vi "Teleop.vi"(10 "Match Info":T1={"Autonomous Elapsed Seconds"=0.0, "TeleOp Elapsed Seconds"=0.0, "Disabled Elapsed Seconds"=0.0, "Visited Autonomous"=FALSE, "Visited TeleOp"=FALSE, "Visited Disabled"=FALSE, "Autonomous Settings"={"Autonomous Style"=enum."Independent", "VI Refnum"=refnum}}, 11 "Call Context":T2) -> ()   [LabVIEW 2016]
doc: "This VI is called for each TeleOp packet received from the DS where the robot is not disabled. It is often used to read from the joysticks and update I/O or to update setpoints for timed control loops. It should complete and return within 20 milliseconds or it may miss DS packets."
uses:
  <vilib>/Rock Robotics/WPI/DriverStation/WPI_DriverStationDerivedRobotMode.ctl
  <vilib>/Rock Robotics/WPI/DriverStation/WPI_DriverStationMatch Info.ctl
  <vilib>/Rock Robotics/WPI/Solenoid/WPI_SolenoidValue.ctl
  <vilib>/Rock Robotics/WPI/Utilities/WPI_GetSetVariantRefNum.vi
  <vilib>/Rock Robotics/WPI/Solenoid/WPI_SolenoidSetEnum.vi
panel:
  out "Gyro Angle":dbl format="%#_13g"
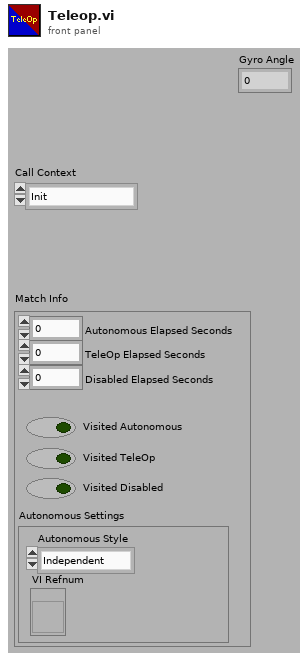
[diagram p1: front panel]
types:
  T1 = typedef "WPI_DriverStationMatch Info.ctl" = cluster{"Autonomous Elapsed Seconds":dbl, "TeleOp Elapsed Seconds":dbl, "Disabled Elapsed Seconds":dbl, "Visited Autonomous":bool, "Visited TeleOp":bool, "Visited Disabled":bool, "Autonomous Settings":cluster{"Autonomous Style":enum16{"Iterative", "Independent"}, "VI Refnum":refnum<vi>}}
  T2 = typedef "WPI_DriverStationDerivedRobotMode.ctl" = enum16{"Init", "Execute", "Stop"}
  T3 = typedef "WPI_SolenoidValue.ctl" = enum16{"Off", "On", "Forward", "Reverse"}
  T4 = typedef "WPI_AccelerometerDevRef.ctl" = cluster{"DevStatus":errorcluster, "Scaling":T5, "Analog Channels":T6, "I2C Bus":T8, "SPI Bus":T9, "Accel Range":T10, "ADXL Axes":T11, "Handle":i32, "Device Address":u8, "Accel Type":enum16{"Analog", "ADXL345 I2C", "ADXL345 SPI", "Internal", "ADXL362 SPI"}}
  T5 = typedef "WPI_AccelerometerScaling.ctl" = cluster{"Gain (VoltsPerG)":dbl, "Center Voltage":dbl}
  T6 = typedef "WPI_AccelerometerAnalogChannels.ctl" = cluster{"X-Axis":T7, "Y-Axis":T7, "Z-Axis":T7}
  T7 = typedef "FPGA_AIChannel.ctl" = enum8{"AI 0", "AI 1", "AI 2", "AI 3", "AI MXP 0", "AI MXP 1", "AI MXP 2", "AI MXP 3", "Invalid"}
  T8 = typedef "i2c_bus.ctl" = enum16{"I2C On-Board", "I2C MXP", "Invalid"}
  T9 = typedef "spi_bus.ctl" = enum16{"SPI On-Board, CS0", "SPI On-Board, CS1", "SPI On-Board, CS2", "SPI On-Board, CS3", "SPI MXP", "Invalid"}
  T10 = typedef "ADXL345 Range.ctl" = u8
  T11 = typedef "WPI_AccelerometerADXL345 Axes.ctl" = cluster{"X-Axis":bool, "Y-Axis":bool, "Z-Axis":bool}
  T12 = cluster{"X-Axis":dbl, "Y-Axis":dbl, "Z-Axis":dbl}
  T13 = typedef "WPI_GyroDevRef.ctl" = cluster{"DevStatus":errorcluster, "Analog Channel":T7, "Offset":dbl, "Gain (VoltsPerDegree/Second)":dbl, "Gyro Type":enum16{"Analog", "XRS450"}, "Handle":i32, "SPI Bus":T9, "Device Found":bool, "Sample Rate":dbl, "Calibrate On Open":bool}
  T14 = typedef "WPI_JoystickDevRef.ctl" = cluster{"Device":T15}
  T15 = typedef "WPI_JoystickDeviceEnum.ctl" = enum16{"USB 0", "USB 1", "USB 2", "USB 3", "USB 4", "USB 5"}
  T16 = typedef "WPI_MotorControlDeviceRef.ctl" = cluster{"DeviceStatus":errorcluster, "Type":T17, "PWM":cluster{"PWM Channel":T18, "DeadBand":T19}, "CAN":cluster{"Device Number":u8, "SetOutput VI Ref":variant, "GetOutput VI Ref":variant, "Enable VI Ref":variant, "Disable VI Ref":variant, "Data":variant}, "Invert":bool}
  T17 = typedef "WPI_MotorControlType.ctl" = enum16{"PWM", "CAN"}
  T18 = typedef "FPGA_DIOPWMChannel.ctl" = enum8{"PWM 0", "PWM 1", "PWM 2", "PWM 3", "PWM 4", "PWM 5", "PWM 6", "PWM 7", "PWM 8", "PWM 9", "PWM MXP 0", "PWM MXP 1", "PWM MXP 2", "PWM MXP 3", "PWM MXP 4", "PWM MXP 5", "PWM MXP 6", "PWM MXP 7", "PWM MXP 8", "PWM MXP 9", "Invalid"}
  T19 = typedef "WPI_PWMDeadband.ctl" = cluster{"Name":string, "maxPositivePwm":i32, "minPositivePwm":i32, "centerPwm":i32, "maxNegativePwm":i32, "minNegativePwm":i32, "angularRange":u16}
  T20 = typedef "WPI_SolenoidDevRef.ctl" = cluster{"DevStatus":errorcluster, "Pneumatics Control Module":u8, "Forward Solenoid Channel":T21, "Reverse Solenoid Channel":T21}
  T21 = typedef "WPI_SolenoidChannel.ctl" = enum8{"Solenoid 0", "Solenoid 1", "Solenoid 2", "Solenoid 3", "Solenoid 4", "Solenoid 5", "Solenoid 6", "Solenoid 7", "Invalid"}
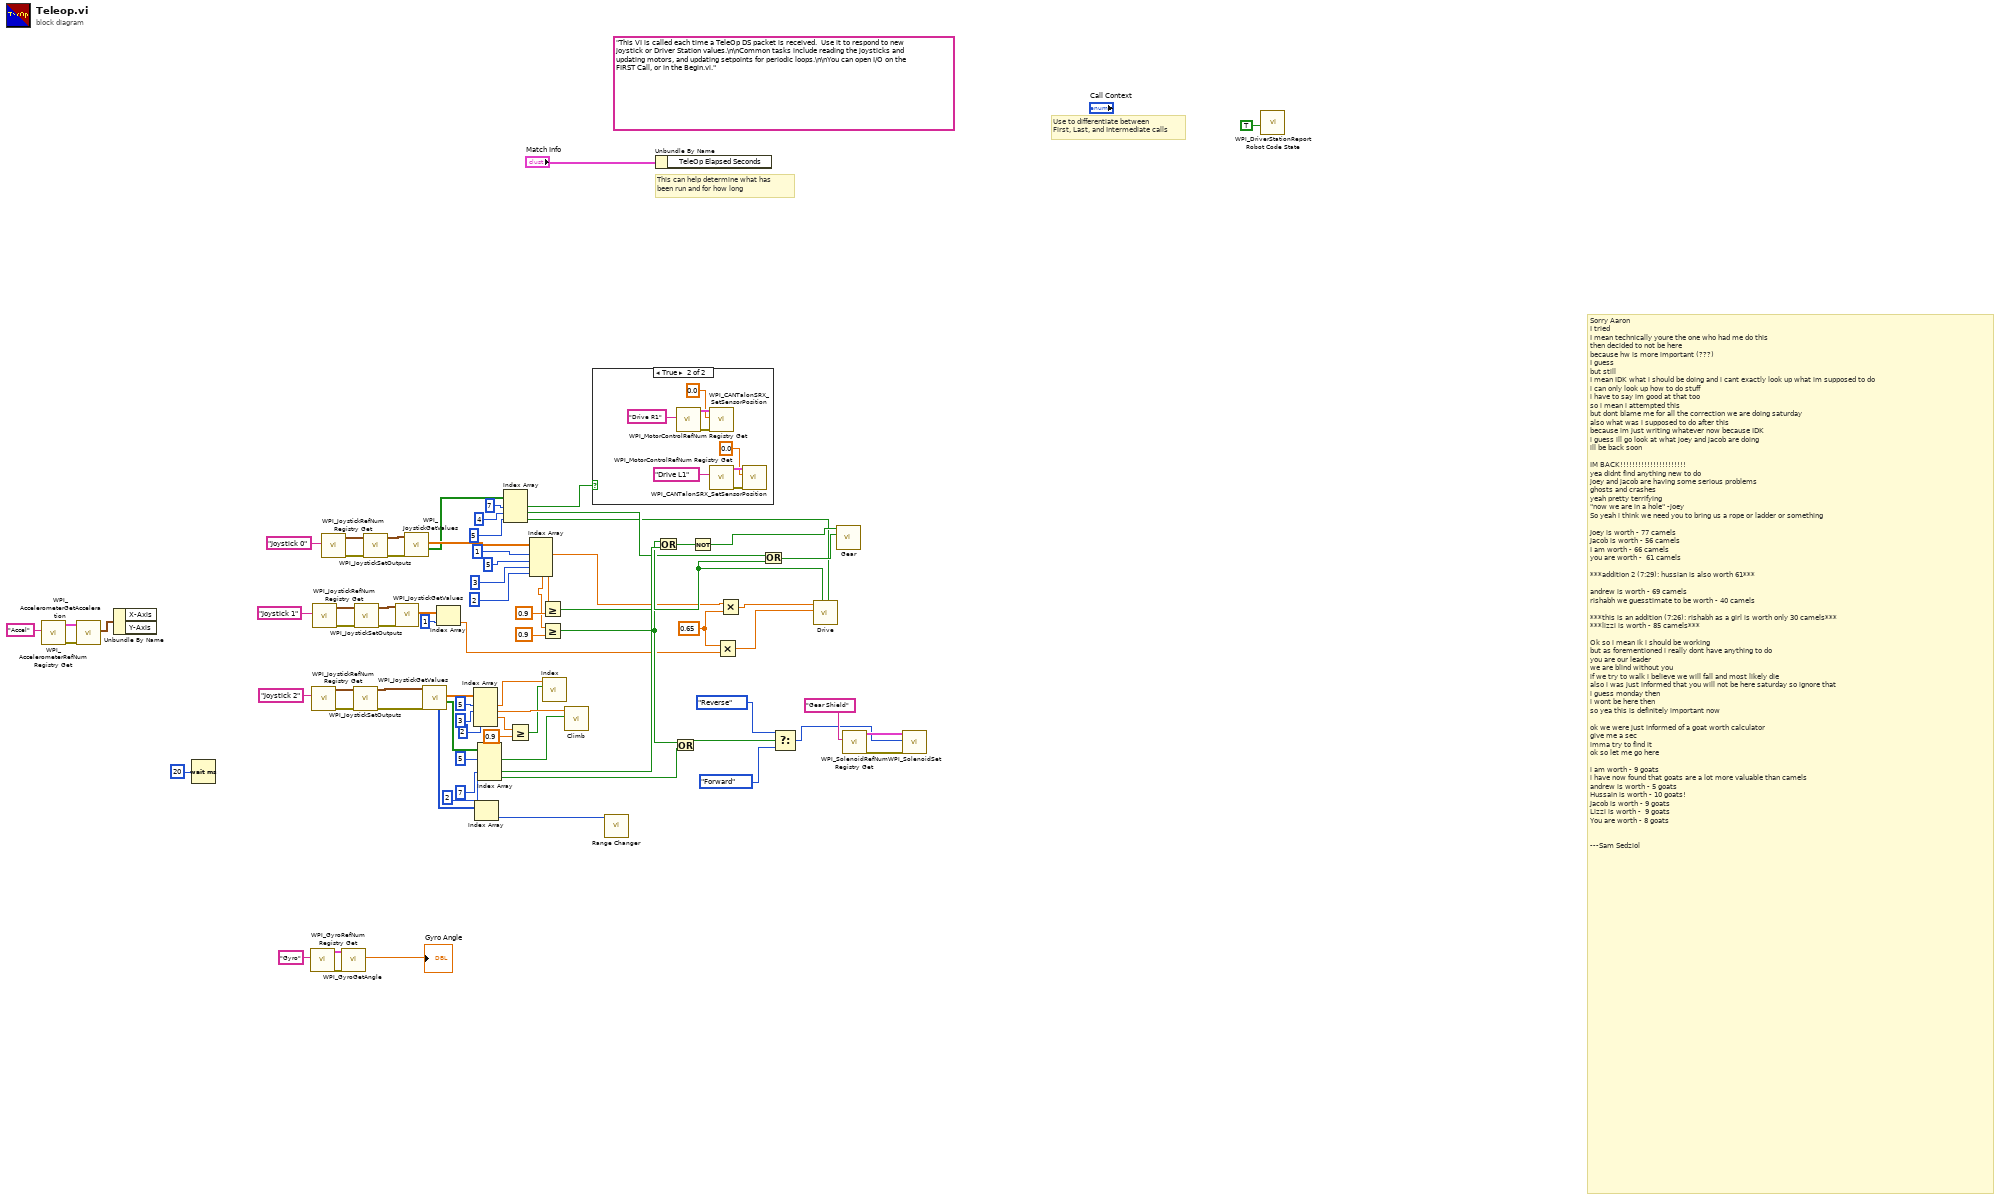
[diagram p0: block diagram]
diagram:
  w1 = 0.65
  (unwired) "This VI is called each time a TeleOp DS packet is received.  Use it to respond to new joystick or Driver Station values.\n\nCommon tasks include reading the joysticks and updating motors, and updating setpoints for periodic loops.\n\nYou can open I/O on the FIRST Call, or in the Begin.vi."
  # "Sorry Aaron\nI tried\nI mean technically youre the one who had me do this\nthen decided to not be here\nbecause hw is more important (???)\nI guess\nbut still\nI mean IDK what i should be doing and i cant exactly look up what im supposed to do\ni can only look up how to do stuff\ni have to say im good at that too\nso i mean i attempted this\nbut dont blame me for all the correction we are doing saturday\nalso what was i supposed to do after this\nbecause im just writing whatever now because IDK\ni guess ill go look at what joey and jacob are doing\nill be back soon\n\nIM BACK!!!!!!!!!!!!!!!!!!!!!!\nyea didnt find anything new to do\njoey and jacob are having some serious problems\nghosts and crashes\nyeah pretty terrifying\n\"now we are in a hole\" -joey\nSo yeah i think we need you to bring us a rope or ladder or something\n\nJoey is worth - 77 camels\nJacob is worth - 56 camels\nI am worth - 66 camels\nyou are worth -  61 camels \n\n***addition 2 (7:29): hussian is also worth 61***\n\nandrew is worth - 69 camels\nrishabh we guesstimate to be worth - 40 camels\n\n***this is an addition (7:26): rishabh as a girl is worth only 30 camels***\n***lizzi is worth - 85 camels***\n\nOk so i mean ik i should be working\nbut as forementioned i really dont have anything to do\nyou are our leader\nwe are blind without you\nif we try to walk i believe we will fall and most likely die\nalso i was just informed that you will not be here saturday so ignore that\ni guess monday then\ni wont be here then\nso yea this is definitely important now\n\nok we were just informed of a goat worth calculator\ngive me a sec \nimma try to find it\nok so let me go here\n\ni am worth - 9 goats\ni have now found that goats are a lot more valuable than camels\nandrew is worth - 5 goats\nHussain is worth - 10 goats! \nJacob is worth - 9 goats\nLizzi is worth -  9 goats\nYou are worth - 8 goats\n\n\n---Sam Sedziol"
  # "Use to differentiate between\nFirst, Last, and Intermediate calls"
  # "This can help determine what has\nbeen run and for how long"
  n1 = call <vilib>:"WPI_AccelerometerRefNum Registry Get.vi"("refnum name"="Accel") -> ("error out"=w23:errorcluster, "AccelerometerDevRef"=w22:T4)  [unwired: 9 in]
  n2 = call <vilib>:"WPI_AccelerometerGetAcceleration.vi"("error in"=w23, "AccelerometerDevRef"=w22) -> ("Accelerations"=w24:T12)  [unwired: 7 in, 2 out]
  n3 = Unbundle By Name(w24) -> ()  [unwired: 2 out]
  n4 = Wait (ms)(milliseconds to wait=u32 20) -> ()  [unwired: 1 out]
  n5 = call <vilib>:"WPI_GyroRefNum Registry Get.vi"("refnum name"="Gyro") -> ("error out"=w63:errorcluster, "GyroDevRef"=w62:T13)  [unwired: 9 in]
  n6 = call <vilib>:"WPI_JoystickRefNum Registry Get.vi"("refnum name"="Joystick 2") -> ("error out"=w17:errorcluster, "JoystickDevRef"=w20:T14)  [unwired: 1 in, 8 out]
  n7 = call <vilib>:"WPI_JoystickRefNum Registry Get.vi"("refnum name"="Joystick 1") -> ("error out"=w11:errorcluster, "JoystickDevRef"=w9:T14)  [unwired: 1 in, 8 out]
  n8 = call <vilib>:"WPI_JoystickRefNum Registry Get.vi"("refnum name"="Joystick 0") -> ("error out"=w14:errorcluster, "JoystickDevRef"=w16:T14)  [unwired: 1 in, 8 out]
  n9 = call <vilib>:"WPI_GyroGetAngle.vi"("error in"=w63, "GyroDevRef"=w62) -> ("Angle"=→"Gyro Angle":dbl)  [unwired: 5 in, 4 out]
  n10 = call <vilib>:"WPI_JoystickSetOutputs.vi"("error in (no error)"=w17, "JoystickDevRef"=w20) -> ("error out"=w18:errorcluster, "JoystickDevRef"=w19:T14)  [unwired: 8 in]
  n11 = call <vilib>:"WPI_JoystickSetOutputs.vi"("error in (no error)"=w11, "JoystickDevRef"=w9) -> ("error out"=w12:errorcluster, "JoystickDevRef"=w10:T14)  [unwired: 8 in]
  n12 = call <vilib>:"WPI_JoystickSetOutputs.vi"("error in (no error)"=w14, "JoystickDevRef"=w16) -> ("error out"=w13:errorcluster, "JoystickDevRef"=w15:T14)  [unwired: 8 in]
  n13 = call <vilib>:"WPI_JoystickGetValues.vi"("error in (no error)"=w12, "JoystickDevRef"=w10) -> ("Axes"=w7:dbl[])  [unwired: 5 in, 4 out]
  n14 = call <vilib>:"WPI_JoystickGetValues.vi"("error in (no error)"=w13, "JoystickDevRef"=w15) -> ("Buttons"=w72:bool[], "Axes"=w76:dbl[])  [unwired: 5 in, 3 out]
  n15 = call <vilib>:"WPI_JoystickGetValues.vi"("error in (no error)"=w18, "JoystickDevRef"=w19) -> ("Buttons"=w73:bool[], "Axes"=w74:dbl[], "POVs"=w51:i16[])  [unwired: 5 in, 2 out]
  n16 = Index Array(array=w7, index=1) -> (element=w2:dbl)
  n17 = Index Array(array=w74, index #1=5 ("index"), index #2=3 ("index"), index #3=2 ("index")) -> (element #1=w59:dbl, element #2=w68:dbl, element #3=w27:dbl)  [unwired: 1 in, 1 out]
  n18 = Index Array(array=w51) -> (element=w50:i16)  [unwired: 1 in]
  n19 = Index Array(array=w73, index #1=5 ("index"), index #3=7 ("index"), index #4=2) -> (element #1=w56:bool, element #3=w57:bool, element #4=w39:bool)  [unwired: 1 in, 1 out]
  n20 = Index Array(array=w72, index #1=7 ("index"), index #2=4 ("index"), index #3=5 ("index")) -> (element #1=w70:bool, element #2=w31:bool, element #3=w29:bool)
  n21 = Greater Or Equal?(x=w27, y=0.9) -> (x >= y?=w25:bool)
  n22 = Index Array(array=w76, index #1=1 ("index"), index #2=5 ("index"), index #3=3 ("index"), index #4=2 ("index")) -> (element #1=w5:dbl, element #3=w38:dbl, element #4=w33:dbl)  [unwired: 1 out]
  n23 = Greater Or Equal?(x=w38, y=0.9) -> (x >= y?=w34:bool)
  n24 = Greater Or Equal?(x=w33, y=0.9) -> (x >= y?=w32:bool)
  n25 = call "Index.vi"("Shoot"=w25, "Output"=w59) -> ()  [unwired: 10 in]
  n26 = call "Climb.vi"("Backwards?"=w56, "Effort"=w68) -> ()  [unwired: 10 in]
  n27 = case shown="True" w70 {
    frame False {
    }
    frame True {
      n28 = call <vilib>:"WPI_MotorControlRefNum Registry Get.vi"("refnum name"="Drive R1") -> ("error out"=w82:errorcluster, "MotorControlDevRef"=w81:T16)  [unwired: 9 in]
      n29 = call <vilib>:"WPI_CANTalonSRX_SetSensorPosition.vi"("error in (no error)"=w82, "New Sensor Position"=0.0, "CAN Talon SRX Ref"=w81) -> ()  [unwired: 7 in, 2 out]
      n30 = call <vilib>:"WPI_MotorControlRefNum Registry Get.vi"("refnum name"="Drive L1") -> ("error out"=w84:errorcluster, "MotorControlDevRef"=w85:T16)  [unwired: 9 in]
      n31 = call <vilib>:"WPI_CANTalonSRX_SetSensorPosition.vi"("error in (no error)"=w84, "New Sensor Position"=0.0, "CAN Talon SRX Ref"=w85) -> ()  [unwired: 7 in, 2 out]
    }
  }
  n32 = call "Range Changer.vi"("POV"=w50) -> ()  [unwired: 10 in, 1 out]
  n33 = Unbundle By Name("Match Info") -> ()  [unwired: 1 out]
  n34 = Or(x=w32, y=w57) -> (x .or. y?=w64:bool)
  n35 = Or(x=w32, y=w39) -> (x .or. y?=w40:bool)
  n36 = Not(x=w64) -> (.not. x?=w54:bool)
  n37 = Multiply(x=w1, y=w2) -> (x*y=w3:dbl)
  n38 = Multiply(x=w5, y=w1) -> (x*y=w4:dbl)
  n39 = Or(x=w31, y=w34) -> (x .or. y?=w53:bool)
  n40 = Select(t=WPI_SolenoidValue."Reverse" ("Value"), s=w40, f=WPI_SolenoidValue."Forward" ("Value")) -> (s? t:f=w43:T3)
  n41 = call "Drive.vi"("SwitchDir"=w29, "Slow?"=w34, "Drive R"=w3, "Drive L"=w4) -> ()  [unwired: 8 in]
  n42 = call "Gear.vi"("Gear0?"=w53, "Gear1?"=w54) -> ()  [unwired: 10 in]
  n43 = call <vilib>:"WPI_SolenoidRefNum Registry Get.vi"("refnum name"="Gear Shield") -> ("error out"=w47:errorcluster, "SolenoidDevRef"=w46:T20)  [unwired: 9 in]
  n44 = call-poly <vilib>:"WPI_SolenoidSet.vi"("error in (no error)"=w47, "Value"=w43, "SolenoidDevRef"=w46) -> ()  [unwired: 7 in, 2 out]
  n45 = call <vilib>:"WPI_DriverStationReport Robot Code State.vi"("TeleOp"=TRUE ("Autonomous")) -> ()  [unwired: 10 in, 1 out]
